vi "esp301 initialize hardware.vi"(7 "Reset (False)":bool, 8 "error in (no error)":errorcluster, 9 "devport":string, 10 "Settings":T1={"devport"="", "Position"={"Axis 1"={"Value"=0.0, "Min"=0.0, "Max"=0.0, "StepSize"=0.0, "Tolerance"=0.0, "ValueActual"=0.0}, "Axis 2"={"Value"=0.0, "Min"=0.0, "Max"=0.0, "StepSize"=0.0, "Tolerance"=0.0, "ValueActual"=0.0}, "Axis 3"={"Value"=0.0, "Min"=0.0, "Max"=0.0, "StepSize"=0.0, "Tolerance"=0.0, "ValueActual"=0.0}}, "Power"={"Axis 1"=enum."off", "Axis 2"=enum."off", "Axis 3"=enum."off"}, "Status"={"Axis 1"=enum."Not referenced", "Axis 2"=enum."Not referenced", "Axis 3"=enum."Not referenced"}, "Backlash"={"Axis 1"={"Value"=0.0, "Min"=0.0, "Max"=0.0, "StepSize"=0.0, "Tolerance"=0.0, "ValueActual"=0.0}, "Axis 2"={"Value"=0.0, "Min"=0.0, "Max"=0.0, "StepSize"=0.0, "Tolerance"=0.0, "ValueActual"=0.0}, "Axis 3"={"Value"=0.0, "Min"=0.0, "Max"=0.0, "StepSize"=0.0, "Tolerance"=0.0, "ValueActual"=0.0}}, "Home"={"Axis 1"={"Value"=0.0, "Min"=0.0, "Max"=0.0, "StepSize"=0.0, "Tolerance"=0.0, "ValueActual"=0.0}, "Axis 2"={"Value"=0.0, "Min"=0.0, "Max"=0.0, "StepSize"=0.0, "Tolerance"=0.0, "ValueActual"=0.0}, "Axis 3"={"Value"=0.0, "Min"=0.0, "Max"=0.0, "StepSize"=0.0, "Tolerance"=0.0, "ValueActual"=0.0}}, "MoveToHardLimit"={"Axis 1"=enum."pos", "Axis 2"=enum."pos", "Axis 3"=enum."pos"}, "relativeMove"={"Axis 1neg"=enum."off", "Axis 2neg"=enum."off", "Axis 3neg"=enum."off", "Axis 1pos"=enum."off", "Axis 2pos"=enum."off", "Axis 3pos"=enum."off"}, "stepsize"={"Value"=0.0, "Min"=0.0, "Max"=0.0, "StepSize"=0.0, "Tolerance"=0.0, "ValueActual"=0.0}, "automotoroff"=enum."off", "ResetBeforeMove"=enum."off", "Enable"={"Axis 1"=enum."on", "Axis 2"=enum."on", "Axis 3"=enum."on"}}, 11 "ESP301 in":refnum<class "ESP301.lvclass">) -> (0 "error out":errorcluster, 2 "VISA resource name out":refnum<visa-resource-name>, 3 "ESP301 out":refnum<class "ESP301.lvclass">)   [LabVIEW 2013, in "ESP301.lvclass"]
uses:
  ESP301.lvclass
  SettingsTypdef.ctl
  OnOffTypeDef.ctl
  status_TypDef.ctl
  Hardware limit.ctl
  ESP301.lvclass/ESP301.ctl
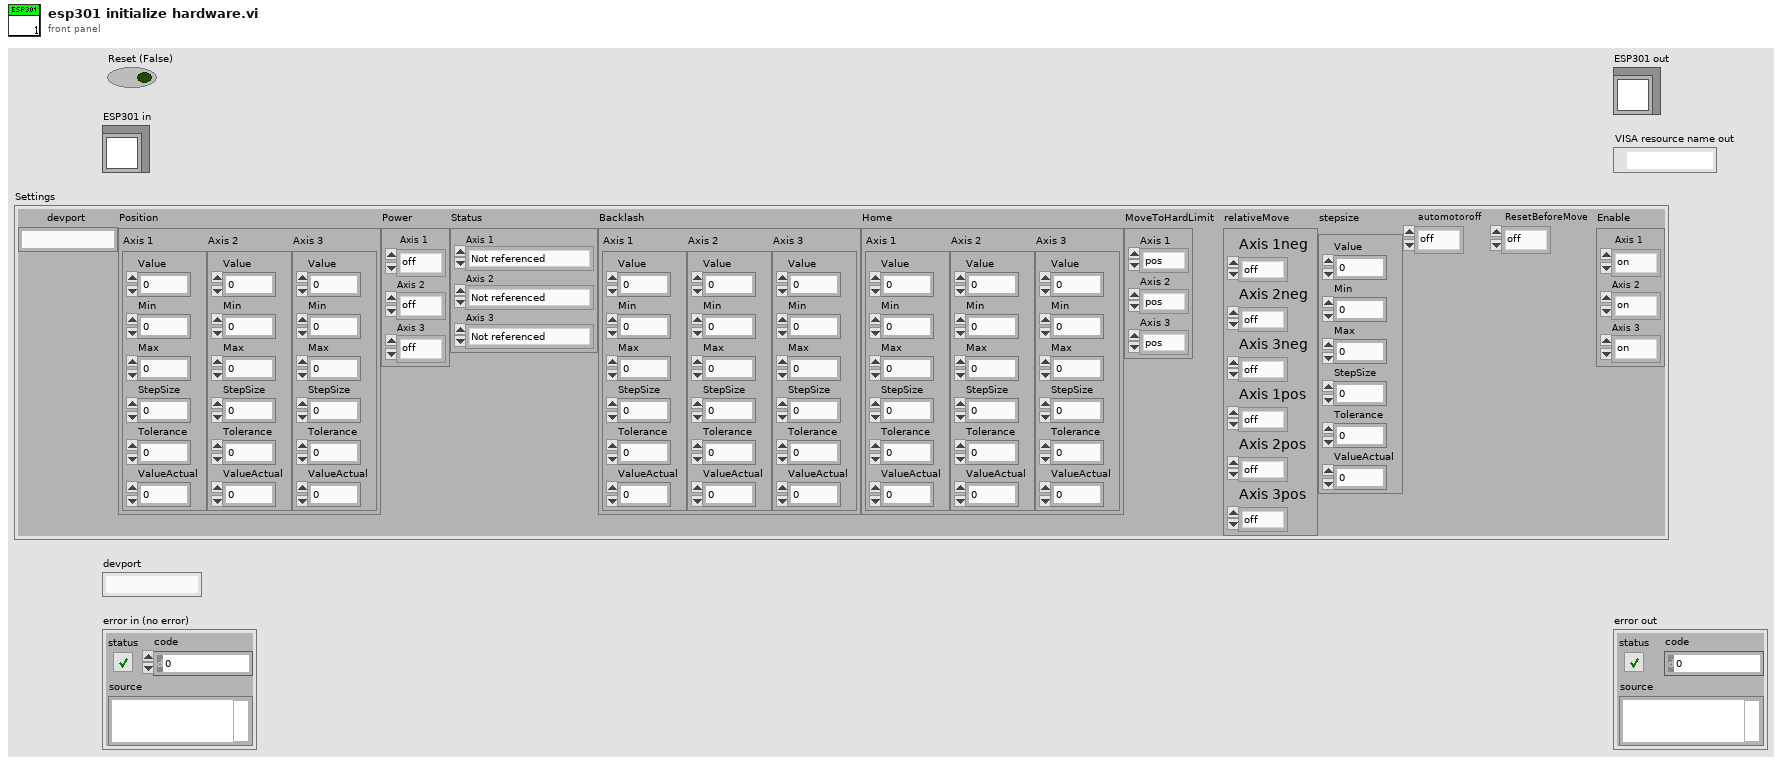
[diagram p1: front panel]
types:
  T1 = typedef "ESP301.lvclass/SettingsTypdef.ctl" = cluster{"devport":string, "Position":cluster{"Axis 1":cluster{"Value":dbl, "Min":dbl, "Max":dbl, "StepSize":dbl, "Tolerance":dbl, "ValueActual":dbl}, "Axis 2":cluster{"Value":dbl, "Min":dbl, "Max":dbl, "StepSize":dbl, "Tolerance":dbl, "ValueActual":dbl}, "Axis 3":cluster{"Value":dbl, "Min":dbl, "Max":dbl, "StepSize":dbl, "Tolerance":dbl, "ValueActual":dbl}}, "Power":cluster{"Axis 1":T2, "Axis 2":T2, "Axis 3":T2}, "Status":cluster{"Axis 1":T3, "Axis 2":T3, "Axis 3":T3}, "Backlash":cluster{"Axis 1":cluster{"Value":dbl, "Min":dbl, "Max":dbl, "StepSize":dbl, "Tolerance":dbl, "ValueActual":dbl}, "Axis 2":cluster{"Value":dbl, "Min":dbl, "Max":dbl, "StepSize":dbl, "Tolerance":dbl, "ValueActual":dbl}, "Axis 3":cluster{"Value":dbl, "Min":dbl, "Max":dbl, "StepSize":dbl, "Tolerance":dbl, "ValueActual":dbl}}, "Home":cluster{"Axis 1":cluster{"Value":dbl, "Min":dbl, "Max":dbl, "StepSize":dbl, "Tolerance":dbl, "ValueActual":dbl}, "Axis 2":cluster{"Value":dbl, "Min":dbl, "Max":dbl, "StepSize":dbl, "Tolerance":dbl, "ValueActual":dbl}, "Axis 3":cluster{"Value":dbl, "Min":dbl, "Max":dbl, "StepSize":dbl, "Tolerance":dbl, "ValueActual":dbl}}, "MoveToHardLimit":cluster{"Axis 1":T4, "Axis 2":T4, "Axis 3":T4}, "relativeMove":cluster{"Axis 1neg":T2, "Axis 2neg":T2, "Axis 3neg":T2, "Axis 1pos":T2, "Axis 2pos":T2, "Axis 3pos":T2}, "stepsize":cluster{"Value":dbl, "Min":dbl, "Max":dbl, "StepSize":dbl, "Tolerance":dbl, "ValueActual":dbl}, "automotoroff":T2, "ResetBeforeMove":T2, "Enable":cluster{"Axis 1":T2, "Axis 2":T2, "Axis 3":T2}}
  T2 = typedef "OnOffTypeDef.ctl" = enum16{"off", "on"}
  T3 = typedef "status_TypDef.ctl" = enum16{"Not referenced", "Homing", "Moving", "Ready"}
  T4 = typedef "Hardware limit.ctl" = enum16{"pos", "neg"}
  T5 = cluster{"Axis 1":cluster{"Value":dbl, "Min":dbl, "Max":dbl, "StepSize":dbl, "Tolerance":dbl, "ValueActual":dbl}, "Axis 2":cluster{"Value":dbl, "Min":dbl, "Max":dbl, "StepSize":dbl, "Tolerance":dbl, "ValueActual":dbl}, "Axis 3":cluster{"Value":dbl, "Min":dbl, "Max":dbl, "StepSize":dbl, "Tolerance":dbl, "ValueActual":dbl}}
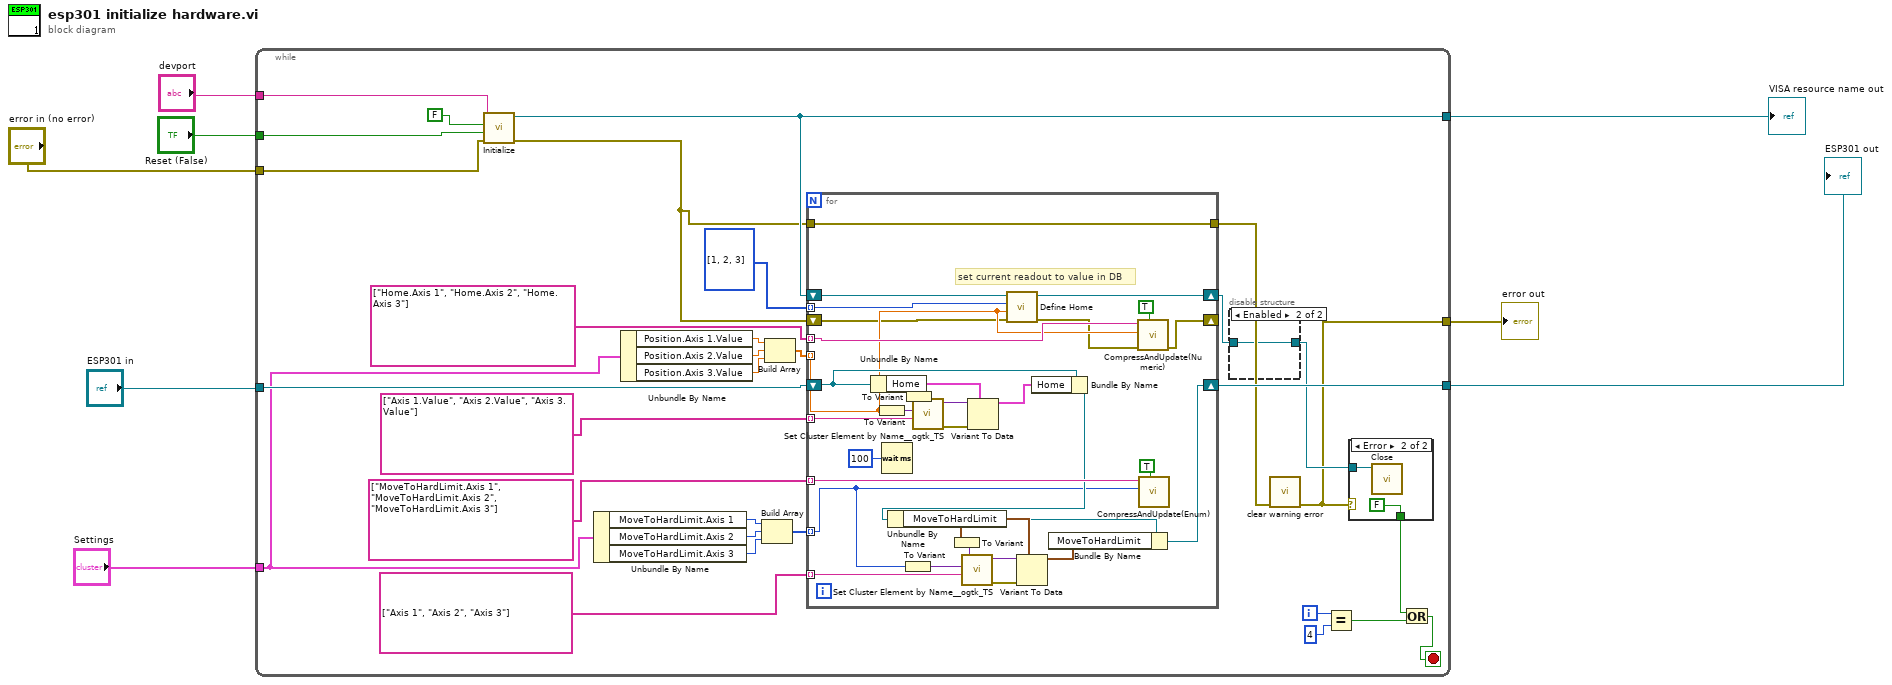
[diagram p0: block diagram]
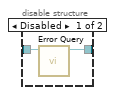
[diagram p2: hidden frame]
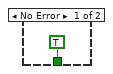
[diagram p3: hidden frame]
diagram:
  n1 = while {
    tunnel: "error in (no error)" -> [w39]
    tunnel: "devport" -> [w37]
    tunnel: "ESP301 in" -> [w31]
    tunnel: [w30] -> w4
    tunnel: [w20] -> w5
    tunnel: "Settings" -> [w19]
    tunnel: [w13] -> w7
    tunnel: "Reset (False)" -> [w9]
    i -> [w18]
    stop <- w15 stop-if-true
    n2 = call "Initialize.vi"("VISA resource name"=w37, "ID Query (True)"=FALSE, "Reset (False)"=w9, "error in (no error)"=w39) -> ("VISA resource name out"=w20:refnum<visa-resource-name>, "error out"=w11:errorcluster)  [unwired: 5 in]
    n3 = Unbundle By Name(w19) -> ("MoveToHardLimit.Axis 1"=w23:T4, "MoveToHardLimit.Axis 2"=w24:T4, "MoveToHardLimit.Axis 3"=w25:T4)
    n4 = Unbundle By Name(w19) -> ("Position.Axis 1.Value"=w35:dbl, "Position.Axis 2.Value"=w34:dbl, "Position.Axis 3.Value"=w33:dbl)
    n5 = Build Array(w23, w24, w25) -> (w22:T4[])
    n6 = Build Array(w35, w34, w33) -> (w32:dbl[])
    n7 = for {
      shift-right: [w67] -> w27
      shift-left: w20 -> [w68]
      tunnel: i32[] [1, 2, 3] -> [w66] mode=indexing
      tunnel: w32 -> [w65] mode=indexing
      shift-right: [w54] -> w30
      shift-left: w31 -> [w72]
      tunnel: string[] ["Axis 1.Value", "Axis 2.Value", "Axis 3.Value"] ("set following Variables (empty = all avriables)") -> [w71] mode=indexing
      tunnel: string[] ["Home.Axis 1", "Home.Axis 2", "Home.Axis 3"] ("set following Variables (empty = all avriables)") -> [w69] mode=indexing
      shift-right: [w62] -> _
      shift-left: w11 -> [w64]
      tunnel: string[] ["MoveToHardLimit.Axis 1", "MoveToHardLimit.Axis 2", "MoveToHardLimit.Axis 3"] ("set following Variables (empty = all avriables)") -> [w60] mode=indexing
      tunnel: w22 -> [w53] mode=indexing
      tunnel: string[] ["Axis 1", "Axis 2", "Axis 3"] ("set following Variables (empty = all avriables)") -> [w52] mode=indexing
      tunnel: w11 -> [w50]
      tunnel: [w50] -> w10
      # "set current readout to value in DB"
      n8 = Unbundle By Name(w72) -> ("Home"=w75:T5)
      n9 = To Variant(anything=w65) -> (Variant=w47:variant)
      n10 = Wait (ms)(milliseconds to wait=u32 100) -> ()  [unwired: 1 out]
      n11 = To Variant(anything=w53) -> (Variant=w48:variant)
      n12 = To Variant(anything=w75) -> (Variant=w46:variant)
      n13 = call "Set Cluster Element by Name__ogtk_TS.vi"("Element Name (\"\": New Element Data Name)"=w71, "New Element Value"=w47, "Cluster"=w46) -> ("error out"=w73:errorcluster, "VCluster out"=w74:variant)  [unwired: 6 in, 1 out]
      n14 = Variant To Data(error in=w73, type=w75, Variant=w74) -> (data=w76:T5)  [unwired: 1 out]
      n15 = call "Define Home.vi"("error in (no error)"=w64, "Home Position (0 units)"=w65, "Axis (1)"=w66, "VISA resource name"=w68) -> ("error out"=w63:errorcluster, "VISA resource name out"=w67:refnum<visa-resource-name>)  [unwired: 2 in]
      n16 = Bundle By Name(cluster=w72, "Home"=w76) -> (w55:refnum<class "ESP301.lvclass">)
      n17 = Unbundle By Name(w55) -> ("MoveToHardLimit"=w57:cluster{"Axis 1":T4, "Axis 2":T4, "Axis 3":T4})
      n18 = To Variant(anything=w57) -> (Variant=w49:variant)
      n19 = call "Set Cluster Element by Name__ogtk_TS.vi"("Element Name (\"\": New Element Data Name)"=w52, "New Element Value"=w48, "Cluster"=w49) -> ("error out"=w59:errorcluster, "VCluster out"=w58:variant)  [unwired: 6 in, 1 out]
      n20 = Variant To Data(error in=w59, type=w57, Variant=w58) -> (data=w56:cluster{"Axis 1":T4, "Axis 2":T4, "Axis 3":T4})  [unwired: 1 out]
      n21 = Bundle By Name(cluster=w55, "MoveToHardLimit"=w56) -> (w54:refnum<class "ESP301.lvclass">)
      n22 = call "CompressAndUpdate(Numeric).vi"("force CVT update (false)"=TRUE ("force CVT update"), "error in"=w63, "Numeric"=w65, "command or variable name"=w69) -> ("error out"=w62:errorcluster)  [unwired: 7 in]
      n23 = call "CompressAndUpdate(Enum).vi"("force CVT update (false)"=TRUE ("force CVT update"), "enum variant"=w53, "command or variable name"=w60) -> ()  [unwired: 8 in, 1 out]
    }
    n24 = disable-structure shown="Enabled" {
      disable-tunnel: w27 -> [w41 w42]
      disable-tunnel: [w40 w42] -> w14
      frame Disabled {
        n25 = call "Error Query.vi"("VISA resource name"=w41) -> ("VISA resource name out"=w40:refnum<visa-resource-name>)  [unwired: 3 in, 3 out]
      }
      frame Enabled {
      }
    }
    n26 = call "clear warning error.vi"("error in"=w10) -> ("error out"=w13:errorcluster)  [unwired: 10 in]
    n27 = Equal?(x=w18, y=4) -> (x = y?=w16:bool)
    n28 = case shown="Error" w13 {
      tunnel: w14 -> [_ w45]
      tunnel: [TRUE FALSE] -> w12
      frame No Error {
      }
      frame Error {
        n29 = call "Close.vi"("VISA resource name"=w45) -> ()  [unwired: 10 in, 1 out]
      }
    }
    n30 = Or(x=w12, y=w16) -> (x .or. y?=w15:bool)
  }
  "error out" <- w7
  "VISA resource name out" <- w5
  "ESP301 out" <- w4
